vi "createState.vi"(8 "error in (no error)":errorcluster, 10 "SWStatus":T1, 11 "MonoStateFactory in":refnum<class "MonoStateFactory.lvclass">) -> (0 "error out":errorcluster, 2 "MonoState.lvclass":refnum<class "MonoState.lvclass">, 3 "MonoStateFactory out":refnum<class "MonoStateFactory.lvclass">)   [LabVIEW 2016, in "MonoStateFactory.lvclass"]
uses:
  MonoStateFactory.lvclass
  MonoStates/MonoState/MonoState.lvclass
  Typedefs/SWStatus.ctl
  MonoStates/OffState/OfflineState.lvclass
  C:/Users/aanania/Documents/ts_monochromator_windows/MonoStates/MonoState/MonoState.lvclass
  MonoStates/ReadyState/ReadySate.lvclass
  MonoStates/SettingUpState/SettingUpState.lvclass
  MonoStates/FaultState/FaultState.lvclass
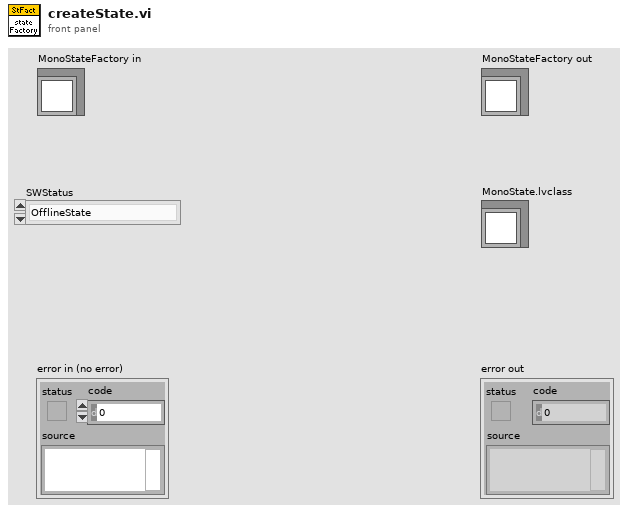
[diagram p1: front panel]
types:
  T1 = typedef "SWStatus.ctl" = enum16{"OfflineState", "ReadyState", "SettingUpState", "FaultState"}
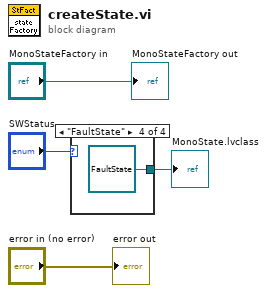
[diagram p0: block diagram]
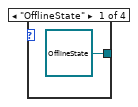
[diagram p2: hidden frame]
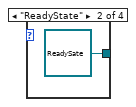
[diagram p3: hidden frame]
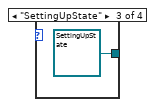
[diagram p4: hidden frame]
diagram:
  n1 = case shown="\"FaultState\"" "SWStatus" {
    tunnel: [refnum<class "OfflineState.lvclass"> refnum ("OfflineState.lvclass") refnum<class "ReadySate.lvclass"> refnum ("ReadySate.lvclass") refnum<class "SettingUpState.lvclass"> refnum ("SettingGratingState.lvclass") refnum<class "FaultState.lvclass"> refnum ("FaultState.lvclass")] -> w1
    frame "OfflineState" {
    }
    frame "ReadyState" {
    }
    frame "SettingUpState" {
    }
    frame "FaultState" {
    }
  }
  "MonoState.lvclass" <- w1
  "error out" <- "error in (no error)"
  "MonoStateFactory out" <- "MonoStateFactory in"
